vi "Parse and Log Multi-Chan Data.vi"(8 "error in (no error)":errorcluster, 10 "MultiChan Variant":variant, 11 "Report Generator in":refnum<class "Report Generator.lvclass">) -> (0 "error out":errorcluster, 3 "Report Generator out":refnum<class "Report Generator.lvclass">)   [LabVIEW 2023, in "Report Generator.lvlib" / "Report Generator.lvclass"]
doc: "Data is easiest passed as a waveform, however, certain dataloggers have memory leaks when logging waveform data, so this takes the waveform data, breaks it down into channel names and data records so that it can be processed without the memory leak. \n\nTherefore the record generator should bundle a group name string, and an array of waveform data to be processed."
uses:
  Library/Report Generator.lvclass
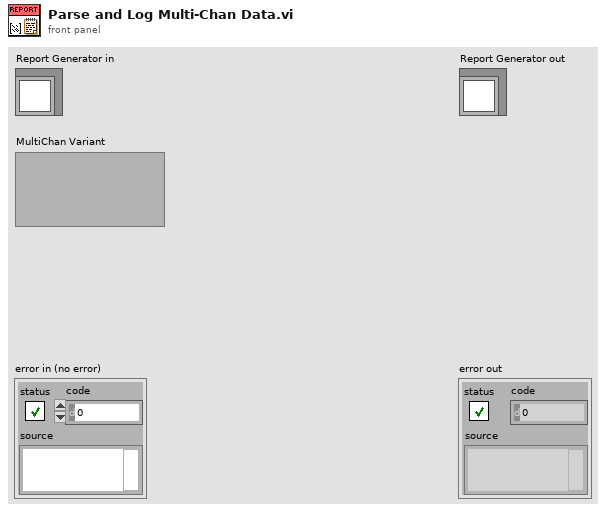
[diagram p1: front panel]
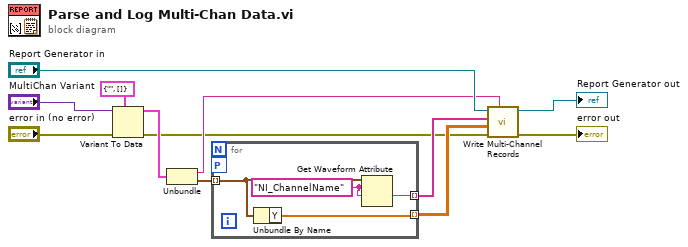
[diagram p0: block diagram]
diagram:
  n1 = Variant To Data(error in="error in (no error)", type=cluster{"Group":string, "Data":waveform(dbl)[]} {"Group"="", "Data"=[]} ("NChanMsg"), Variant="MultiChan Variant") -> (data=w5:cluster{"Group":string, "Data":waveform(dbl)[]}, error out=w1:errorcluster)
  n2 = Unbundle(w5) -> ("Group"=w3:string, "Data"=w4:waveform(dbl)[])
  n3 = for {
    tunnel: w4 -> [w15] mode=indexing
    tunnel: [w16] -> w9 mode=indexing
    tunnel: [w13] -> w8 mode=indexing
    workers-P: _ -> [_]
    w14 = "NI_ChannelName" ("name")
    n4 = Unbundle By Name(w15) -> ("Y"=w16:dbl[])
    n5 = Get Waveform Attribute(5:w14, 6:w14, 7:w15) -> (1:w13:string)  [unwired: 1 in, 3 out]
  }
  n6 = call-dynamic "Write Multi-Channel Records.vi"("Group"=w3, "error in (no error)"=w1, "Data"=w9, "Channels"=w8, "Report Generator in"="Report Generator in") -> ("error out"=→"error out":errorcluster, "Report Generator out"=→"Report Generator out":refnum<class "Report Generator.lvclass">)  [unwired: 5 in]
